vi "Set Cell Column Span.vi"(7 "Range":i32, 8 "error in":errorcluster, 9 "Column":i32, 10 "Row":i32, 11 "SourceGrid in":refnum<class "SourceGrid.lvclass">) -> (0 "error out":errorcluster, 3 "SourceGrid out":refnum<class "SourceGrid.lvclass">)   [LabVIEW 2024, in "SourceGrid.lvlib" / "SourceGrid.lvclass"]
doc: "ColSpan for merge operation, calculated using the current range."
uses:
  SourceGrid.lvclass
  SourceGrid.lvclass/SourceGrid.ctl
  D:/git/Sourcegrid-LabVIEW/dll/SourceGrid.dll
  dll/SourceGrid.dll
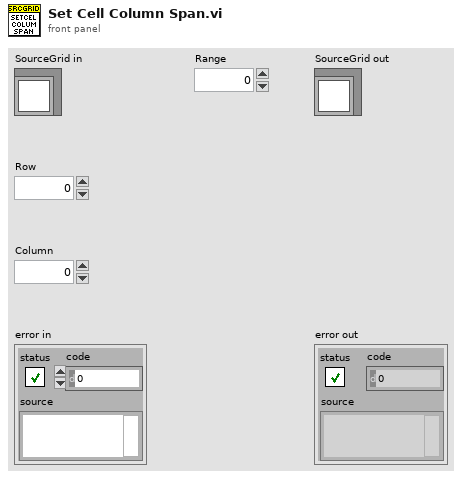
[diagram p1: front panel]
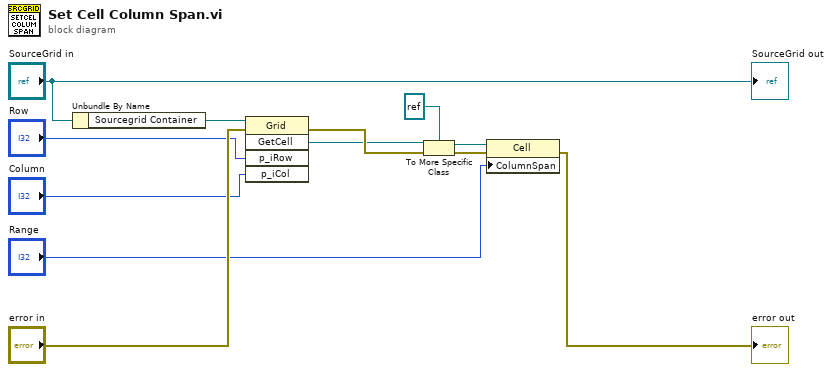
[diagram p0: block diagram]
diagram:
  n1 = Unbundle By Name("SourceGrid in") -> ("Sourcegrid Container"=w11:refnum<k24>)
  n2 = invoke class="Grid" method="GetCell"(reference=w11, error in="error in", "p_iRow"="Row", "p_iCol"="Column") -> (error out=w9:errorcluster, "GetCell"=w2:refnum<k24>)  [unwired: 1 in, 3 out]
  n3 = To More Specific Class(target class=refnum<k24> refnum ("new reference"), reference=w2, error in=w9) -> (specific class reference=w1:refnum<k24>, error out=w6:errorcluster)
  n4 = property class="Cell"(reference=w1, error in=w6, "ColumnSpan"="Range") -> (error out=→"error out":errorcluster)  [unwired: 1 out]
  "SourceGrid out" <- "SourceGrid in"
